vi "SimpleMotorFF_Calculate_NextV_Dt.vi"(8 "dT_Sec":dbl=0.02, 9 "NextVel_SP":dbl, 10 "Vel_SP":dbl, 11 "SIMPLE_MOTOR_FF":T1 {"Ka" format="%13.4f"; "Kv" format="%13.4f"; "Ks" format="%13.4f"}) -> (0 "Error":bool, 3 "FeedForward":dbl)   [LabVIEW 2019, in "Trajectory_Library.lvlib"]
doc: "Calculates the feedforward from the gains and setpoints. This VI calculates the acceleration by using a Linear System and a Linear Plant Inversion Feedforward. These systems are only created upon the first call or when one of the Kv or Ka values change.\n \nInput parameters:\n - SimpleMotorFF - Data structure containing constants\n - Vel_SP -- The current velocity setpoint. (The velocity SP that was used last scan cycle)\n - nextVel_SP -- The next velocity setpoint. (The velocity SP that we are using this scan cycle.)\n - dt_Sec -- Time between velocity setpoints in seconds.\n \nReturns:\n - FeedForward - The computed feedforward.\n - Error -- If TRUE, an error occured calculating the acceleration value."
uses:
  Trajectory_Library.lvlib
  TypeDef/SIMPLE_MOTOR_FF.ctl
  MatBuilder_Create.vi
  LinearSystem_New.vi
  MatrixHelper_Zero.vi
  MatBuilder_Fill.vi
  MatrixHelper_CoerceSize.vi
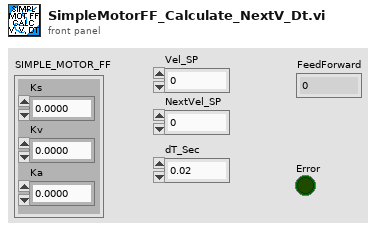
[diagram p1: front panel]
types:
  T1 = typedef "Trajectory_Library.lvlib/SIMPLE_MOTOR_FF.ctl" = cluster{"Ks":dbl, "Kv":dbl, "Ka":dbl}
  T2 = typedef "NI_Matrix.lvlib/RealMatrix.ctl" = dbl[][]
  T3 = typedef "Trajectory_Library.lvlib/LINEAR_PLANT_INV_FF.ctl" = cluster{"m_R":T2, "m_Uff":T2, "m_B":T2, "m_A":T2, "States":i32, "Inputs":i32}
  T4 = typedef "Trajectory_Library.lvlib/LINEAR_SYSTEM.ctl" = cluster{"m_A":T2, "m_B":T2, "m_C":T2, "m_D":T2, "States":i32, "Inputs":i32, "Outputs":i32}
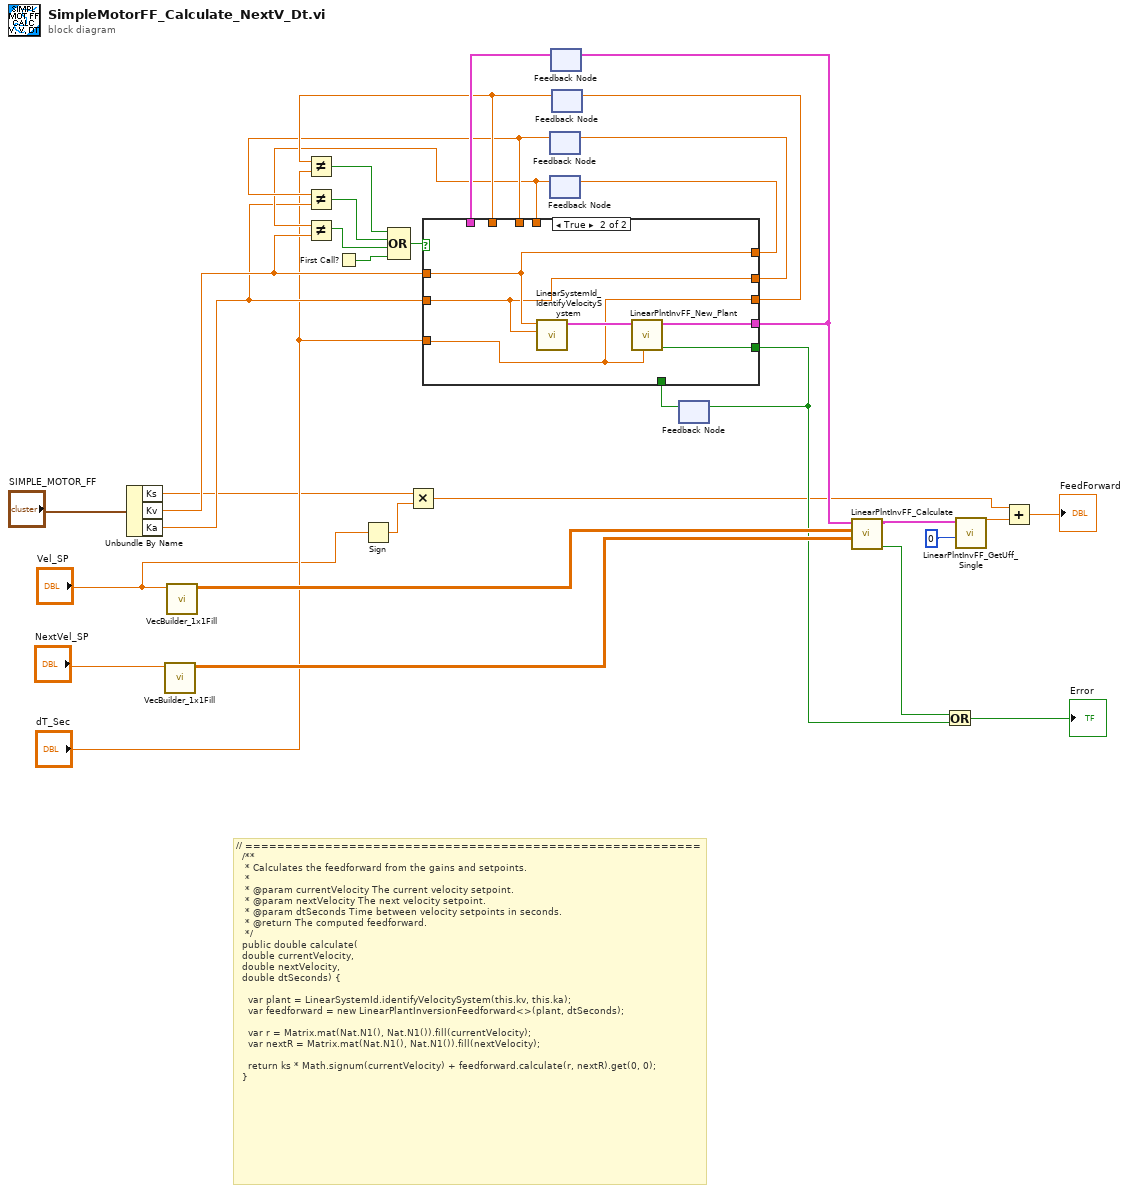
[diagram p0: block diagram]
diagram:
  # "// =========================================================\n  /**\n   * Calculates the feedforward from the gains and setpoints.\n   *\n   * @param currentVelocity The current velocity setpoint.\n   * @param nextVelocity The next velocity setpoint.\n   * @param dtSeconds Time between velocity setpoints in seconds.\n   * @return The computed feedforward.\n   */\n  public double calculate(\n\t\tdouble currentVelocity, \n\t\tdouble nextVelocity, \n\t\tdouble dtSeconds) {\n\n    var plant = LinearSystemId.identifyVelocitySystem(this.kv, this.ka);\n    var feedforward = new LinearPlantInversionFeedforward<>(plant, dtSeconds);\n\n    var r = Matrix.mat(Nat.N1(), Nat.N1()).fill(currentVelocity);\n    var nextR = Matrix.mat(Nat.N1(), Nat.N1()).fill(nextVelocity);\n\n    return ks * Math.signum(currentVelocity) + feedforward.calculate(r, nextR).get(0, 0);\n  }"
  n1 = Unbundle By Name("SIMPLE_MOTOR_FF") -> ("Ks"=w8:dbl, "Kv"=w16:dbl, "Ka"=w15:dbl)
  n2 = call "VecBuilder_1x1Fill.vi"("R0_C0"="NextVel_SP") -> ("output matrix"=w25:T2)  [unwired: 10 in]
  n3 = call "VecBuilder_1x1Fill.vi"("R0_C0"="Vel_SP") -> ("output matrix"=w26:T2)  [unwired: 10 in]
  n4 = First Call?() -> (First Call?: T/F=w13:bool)
  n5 = Sign(1:"Vel_SP") -> (0:w7:dbl)
  n6 = Multiply(x=w8, y=w7) -> (x*y=w6:dbl)
  n7 = feedback #1() -> (w18:dbl)  [unwired: 1 in]
  n8 = Not Equal?(x=w18, y=w15) -> (x != y?=w11:bool)
  n9 = feedback #2() -> (w17:dbl)  [unwired: 1 in]
  n10 = Not Equal?(x=w17, y=w16) -> (x != y?=w12:bool)
  n11 = feedback #3() -> (w29:T3)  [unwired: 1 in]
  n12 = feedback #4() -> (w19:dbl)  [unwired: 1 in]
  n13 = Not Equal?(x=w19, y="dT_Sec") -> (x != y?=w10:bool)
  n14 = Compound Arithmetic op=OR(w10, w11, w12, w13) -> (w30:bool)
  n15 = feedback #5() -> (w20:bool)  [unwired: 1 in]
  n16 = case shown="True" w30 {
    tunnel: [w36 w42] -> w28
    tunnel: w29 -> [w36 _]
    tunnel: w16 -> [_ w41]
    tunnel: [w37 w41] -> w24
    tunnel: w15 -> [_ w39]
    tunnel: "dT_Sec" -> [_ w38]
    tunnel: [w33 w40] -> w21
    tunnel: [w35 w39] -> w23
    tunnel: w17 -> [w37 _]
    tunnel: w18 -> [w35 _]
    tunnel: w19 -> [w34 _]
    tunnel: [w34 w38] -> w22
    tunnel: w20 -> [w33 _]
    frame False {
    }
    frame True {
      n17 = call "LinearSystemId_IdentifyVelocitySystem.vi"("kA"=w39, "kV"=w41) -> ("Linearsystem"=w43:T4)  [unwired: 8 in, 1 out]
      n18 = call "LinearPlntInvFF_New_Plant.vi"("dT_Seconds"=w38, "Plant"=w43) -> ("Error"=w40:bool, "Linear Plnt Inversion FF"=w42:T3)  [unwired: 8 in]
    }
  }
  n19 = feedback-in #1(w23) -> ()
  n20 = feedback-in #2(w24) -> ()
  n21 = feedback-in #3(w28) -> ()
  n22 = feedback-in #4(w22) -> ()
  n23 = feedback-in #5(w21) -> ()
  n24 = call "LinearPlntInvFF_Calculate.vi"("NextR"=w25, "R"=w26, "Input Linear Plant Inv FF"=w28) -> ("Error"=w27:bool, "Output Linear Plant Inv FF"=w2:T3)  [unwired: 6 in, 1 out]
  n25 = Or(x=w27, y=w21) -> (x .or. y?=→"Error":bool)
  n26 = call "LinearPlntInvFF_GetUff_Single.vi"("Row"=0, "Linear Plnt Inversion FF"=w2) -> ("Uff"=w3:dbl)  [unwired: 9 in]
  n27 = Add(x=w6, y=w3) -> (x+y=→"FeedForward":dbl)
